vi "ScratchPad_FindBlocksvi.vi"() -> ()   [LabVIEW 2013, in "Graph.lvclass"]
uses:
  Graph.lvclass
panel:
  out "Array 2":i32[][](array[numeric])
  out "Array":i32[][](array[numeric])
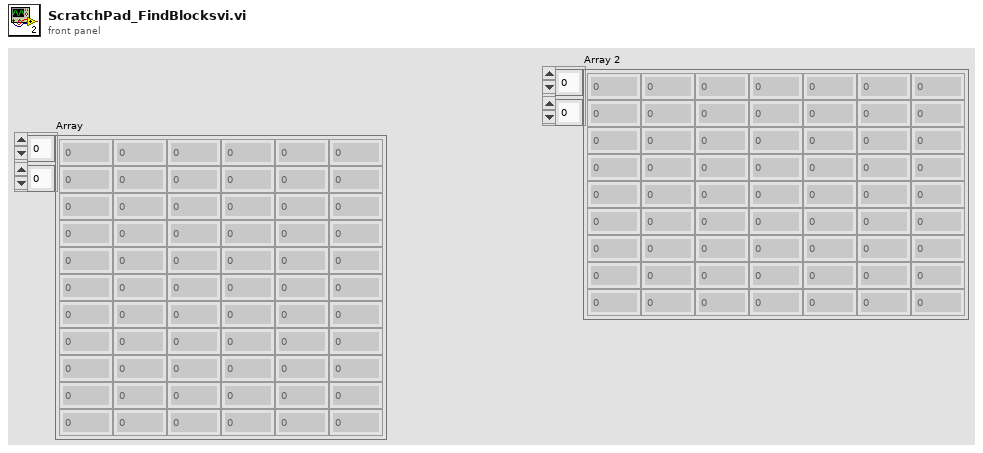
[diagram p1: front panel]
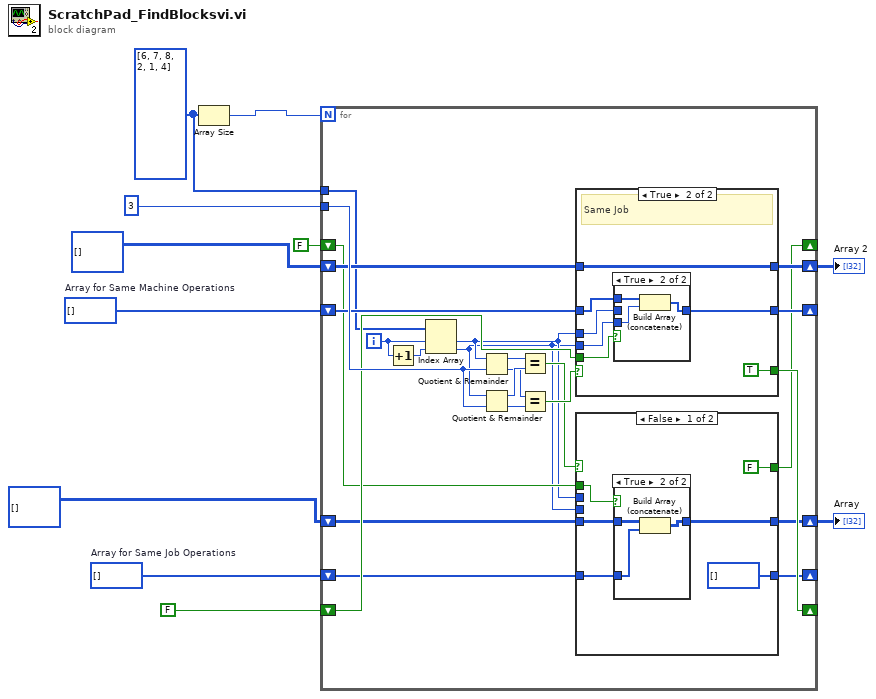
[diagram p0: block diagram]
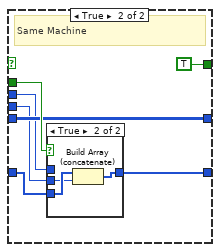
[diagram p3: hidden frame]
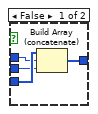
[diagram p4: hidden frame]
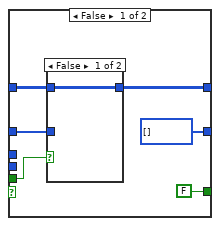
[diagram p5: hidden frame]
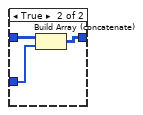
[diagram p6: hidden frame]
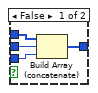
[diagram p7: hidden frame]
diagram:
  w2 = i32[] []  # Array for Same Job Operations
  w4 = i32[] []  # Array for Same Machine Operations
  w5 = i32[] [6, 7, 8, 2, 1, 4] ("array w/ subset deleted")
  n1 = Array Size(array=w5) -> (size(s)=w1:i32)
  n2 = for {
    N: w1 -> [_]
    tunnel: w5 -> [w25]
    tunnel: 3 -> [w35]
    shift-right: [w26] -> w8
    shift-left: i32[][] [] -> [w27]
    shift-right: [w12] -> w9
    shift-left: i32[][] [] -> [w15]
    shift-right: [w28] -> _
    shift-left: FALSE -> [w30]
    shift-right: [w21] -> _
    shift-left: w4 -> [w29]
    shift-right: [w19] -> _
    shift-left: FALSE -> [w20]
    shift-right: [w16] -> _
    shift-left: w2 -> [w18]
    i -> [w24]
    n3 = Increment(x=w24) -> (x+1=w23:i32)
    n4 = Index Array(array=w25, index #1=w24, index #2=w23) -> (element #1=w14:i32, element #2=w13:i32)
    n5 = Quotient & Remainder(x=w14, y=w35) -> (x-y*floor(x/y)=w33:i32, floor(x/y)=w31:i32)
    n6 = Quotient & Remainder(x=w13, y=w35) -> (x-y*floor(x/y)=w34:i32, floor(x/y)=w32:i32)
    n7 = Equal?(x=w33, y=w34) -> (x = y?=w17:bool)
    n8 = Equal?(x=w31, y=w32) -> (x = y?=w22:bool)
    n9 = case shown="True" w22 {
      tunnel: w30 -> [w63 w76]
      tunnel: w29 -> [w61 w75]
      tunnel: [i32[] [] w74] -> w21
      tunnel: [FALSE TRUE] -> w28
      tunnel: w27 -> [w62 w72]
      tunnel: [w60 w72] -> w26
      tunnel: w14 -> [_ w71]
      tunnel: w13 -> [_ w70]
      frame False {
        n10 = case shown="False" w63 {
          tunnel: w62 -> [w66 w69]
          tunnel: w61 -> [_ w68]
          tunnel: [w66 w67] -> w60
          frame False {
          }
          frame True {
            n11 = Build Array (concatenate)(w69, w68) -> (w67:i32[][])
          }
        }
      }
      frame True {
        # "Same Job"
        n12 = case shown="True" w76 {
          tunnel: w75 -> [w80 w83]
          tunnel: [w77 w82] -> w74
          tunnel: w71 -> [w79 _]
          tunnel: w70 -> [w78 w81]
          frame False {
            n13 = Build Array (concatenate)(w80, w79, w78) -> (w77:i32[])
          }
          frame True {
            n14 = Build Array (concatenate)(w83, w81) -> (w82:i32[])
          }
        }
      }
    }
    n15 = case shown="False" w17 {
      tunnel: w20 -> [w39 w52]
      tunnel: w18 -> [w37 w51]
      tunnel: [i32[] [] w50] -> w16
      tunnel: [FALSE TRUE] -> w19
      tunnel: w15 -> [w38 w48]
      tunnel: [w36 w48] -> w12
      tunnel: w14 -> [_ w47]
      tunnel: w13 -> [_ w46]
      frame False {
        n16 = case shown="True" w39 {
          tunnel: w38 -> [w42 w45]
          tunnel: w37 -> [_ w44]
          tunnel: [w42 w43] -> w36
          frame False {
          }
          frame True {
            n17 = Build Array (concatenate)(w45, w44) -> (w43:i32[][])
          }
        }
      }
      frame True {
        # "Same Machine"
        n18 = case shown="True" w52 {
          tunnel: w51 -> [w56 w59]
          tunnel: [w53 w58] -> w50
          tunnel: w47 -> [w55 _]
          tunnel: w46 -> [w54 w57]
          frame False {
            n19 = Build Array (concatenate)(w56, w55, w54) -> (w53:i32[])
          }
          frame True {
            n20 = Build Array (concatenate)(w59, w57) -> (w58:i32[])
          }
        }
      }
    }
  }
  "Array" <- w9
  "Array 2" <- w8
